vi "Number_of_Windows.vi"() -> ()   [LabVIEW 2020]
panel:
  out "Number_of_Windows":i64
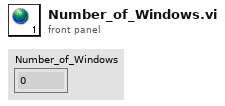
[diagram p1: front panel]
diagram:
